vi "Stop Helper Loops.vi"(8 "error in (no error)":errorcluster, 11 "Helper Loop In":refnum<class "Helper Loop.lvclass">) -> (0 "error out":errorcluster, 3 "Helper Loop Out":refnum<class "Helper Loop.lvclass">)   [LabVIEW 2020, in "Helper Loop.lvclass"]
doc: "This method stops the helper loop.The Helper Action may stop the helper loop by throwing an error. If this has happened prior to calling this method, a time out will occur."
uses:
  Helper Loop.lvclass
  Process/Process.lvclass
  <vilib>/Utility/error.llb/Error Cluster From Error Code.vi
  <vilib>/ErrorRing/Error Ring.xnode
  Process/Public/Lifecycle/API Mode.ctl
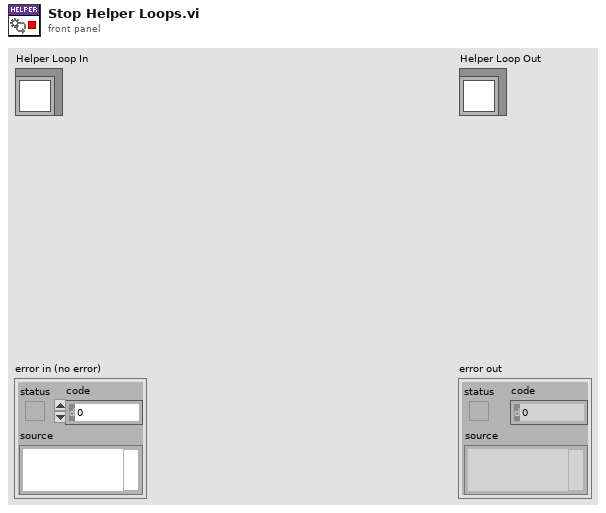
[diagram p1: front panel]
types:
  T1 = typedef "Process.lvclass/API Mode.ctl" = enum16{"Send Message", "Handle Message"}
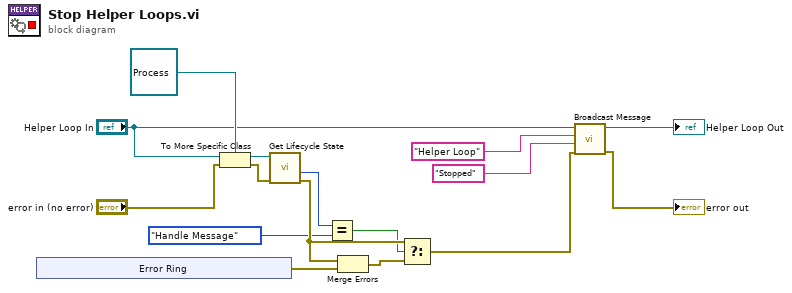
[diagram p0: block diagram]
diagram:
  n1 = xnode "Error Ring"() -> ("error out"=w9:errorcluster)
  n2 = To More Specific Class(target class=refnum<class "Process.lvclass"> refnum ("Process Out"), reference="Helper Loop In", error in="error in (no error)") -> (specific class reference=w15:refnum<class "Process.lvclass">, error out=w13:errorcluster)
  n3 = call "Get Lifecycle State.vi"("error in (no error)"=w13, "Process In"=w15) -> ("error out"=w12:errorcluster, "API Mode"=w11:T1)  [unwired: 6 in, 2 out]
  n4 = Equal?(x=w11, y=API_Mode."Handle Message") -> (x = y?=w2:bool)
  n5 = Merge Errors(w12, w9) -> (w10:errorcluster)
  n6 = Select(t=w12, s=w2, f=w10) -> (s? t:f=w5:errorcluster)
  n7 = call-dynamic "Broadcast Message.vi"("error in (no error)"=w5, "Message Data"="Stopped" ("Message"), "Message"="Helper Loop", "Helper Loop in"="Helper Loop In") -> ("error out"=→"error out":errorcluster, "Helper Loop out"=→"Helper Loop Out":refnum<class "Helper Loop.lvclass">)  [unwired: 6 in]
